vi "Currentl Fork Level.vi"(9 "Right":bool) -> (1 "Level":dbl)   [LabVIEW 2014]
uses:
  v9/Robot Global Data.vi
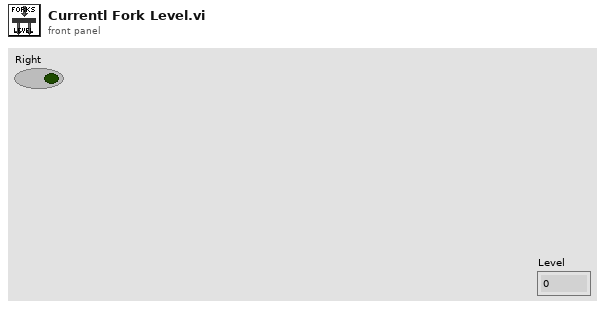
[diagram p1: front panel]
types:
  T1 = typedef "WPI_MotorControlDeviceRef.ctl" = cluster{"DeviceStatus":errorcluster, "Type":T2, "PWM":cluster{"Controller":T3, "PWM Channel":T4, "DeadBand":T5}, "CAN":cluster{"Device Number":u8, "Control Mode":T6, "Semaphore":T7, "Max Vout":dbl, "TalonSRX Control Mode":T8}, "Invert":bool, "TransformRef":T9, "InvTransformRef":T9}
  T2 = typedef "WPI_MotorControlType.ctl" = enum16{"PWM", "CAN", "CANTalonSRX"}
  T3 = typedef "FPGA_TypedefDigitalModule.ctl" = enum16{"Controller 1"}
  T4 = typedef "FPGA_DIOPWMChannel.ctl" = enum8{"PWM 0", "PWM 1", "PWM 2", "PWM 3", "PWM 4", "PWM 5", "PWM 6", "PWM 7", "PWM 8", "PWM 9", "PWM MXP 0", "PWM MXP 1", "PWM MXP 2", "PWM MXP 3", "PWM MXP 4", "PWM MXP 5", "PWM MXP 6", "PWM MXP 7", "PWM MXP 8", "PWM MXP 9", "Invalid"}
  T5 = typedef "WPI_PWMDeadband.ctl" = cluster{"Name":string, "maxPositivePwm":i32, "minPositivePwm":i32, "centerPwm":i32, "maxNegativePwm":i32, "minNegativePwm":i32, "angularRange":u16}
  T6 = typedef "WPI_CANJaguar_ControlMode.ctl" = enum8{"Percent VBus", "Current", "Speed", "Position", "Voltage"}
  T7 = typedef "Semaphore RefNum" = refnum<k1>
  T8 = typedef "WPI_CANTalonSRX_APIControlMode.ctl" = enum8{"Percent VBus", "Speed", "Position", "Slave", "Unchanged / Invalid"}
  T9 = typedef "WPI_PWMTransform_ConPane.ctl" = refnum<vi>
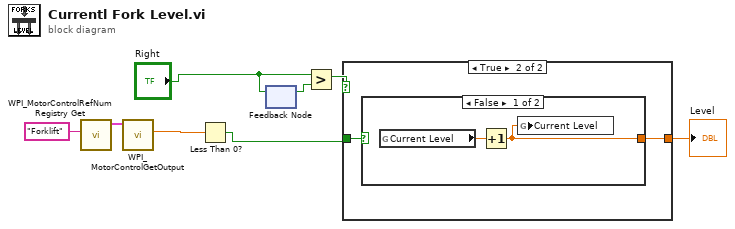
[diagram p0: block diagram]
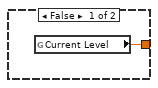
[diagram p2: hidden frame]
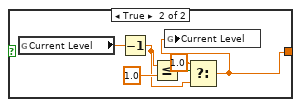
[diagram p3: hidden frame]
diagram:
  n1 = call <vilib>:"WPI_MotorControlRefNum Registry Get.vi"("refnum name"="Forklift") -> ("MotorControlDevRef"=w8:T1)  [unwired: 9 in, 1 out]
  n2 = call <vilib>:"WPI_MotorControlGetOutput.vi"("MotorControlDevRef"=w8) -> ("Output"=w5:dbl)  [unwired: 8 in, 2 out]
  n3 = Less Than 0?(x=w5) -> (x < 0?=w4:bool)
  n4 = feedback-in #1("Right") -> ()
  n5 = feedback #1() -> (w2:bool)  [unwired: 1 in]
  n6 = Greater?(x="Right", y=w2) -> (0:w3:bool)
  n7 = case shown="True" w3 {
    tunnel: [w9 w11] -> w6
    tunnel: w4 -> [_ w10]
    frame False {
      n8 = global read "Robot Global Data.vi" "Current Level"() -> (w9:dbl)
    }
    frame True {
      n9 = case shown="False" w10 {
        tunnel: [w12 w16] -> w11
        frame False {
          n10 = global read "Robot Global Data.vi" "Current Level"() -> (w13:dbl)
          n11 = Increment(x=w13) -> (x+1=w12:dbl)
          n12 = global write "Robot Global Data.vi" "Current Level"(w12) -> ()
        }
        frame True {
          n13 = global read "Robot Global Data.vi" "Current Level"() -> (w19:dbl)
          n14 = Decrement(x=w19) -> (x-1=w15:dbl)
          n15 = Less Or Equal?(x=w15, y=1.0) -> (x <= y?=w17:bool)
          n16 = Select(t=1.0, s=w17, f=w15) -> (s? t:f=w16:dbl)
          n17 = global write "Robot Global Data.vi" "Current Level"(w16) -> ()
        }
      }
    }
  }
  "Level" <- w6
